vi "ProduceCharString.vi"(2 "CharToBeProduce":string, 3 "NumOfStr":u32) -> (0 "ResultStr":string)   [LabVIEW 2011]
panel:
  # "产生一个由所给字符（串）和数量参数决定的连续字符串，比如给出NumOfStr=5 CharToBeProduce=a  则产生\"aaaaa\""
  # "子VI作用是将命令打包成规定的数据格式，输入参数包括模块名称（或模块代号）和命令"
  # "输入"
  # "输出"
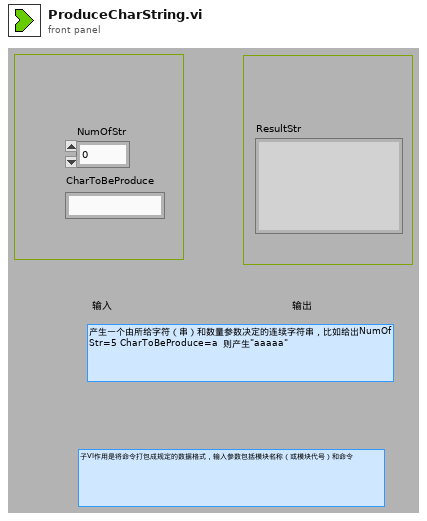
[diagram p1: front panel]
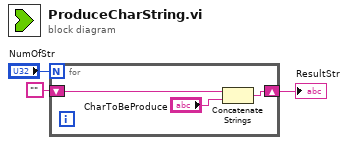
[diagram p0: block diagram]
diagram:
  n1 = for {
    N: "NumOfStr" -> [_]
    shift-right: [w4] -> w1
    shift-left: "" -> [w6]
    n2 = Concatenate Strings(w6, "CharToBeProduce") -> (w4:string)
  }
  "ResultStr" <- w1
